vi "Array 1.vi"(8 "Error In":errorcluster) -> (0 "Error Out":errorcluster)   [LabVIEW 2014]
uses:
  <vilib>/Aledyne-TSXperts/Arduino Compatible Compiler for LabVIEW/addons/Arduino SoftwareSerial Wrapper/Arduino SoftwareSerial Wrapper.lvlib
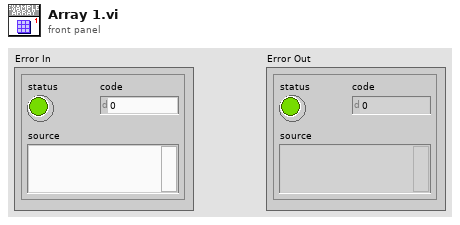
[diagram p1: front panel]
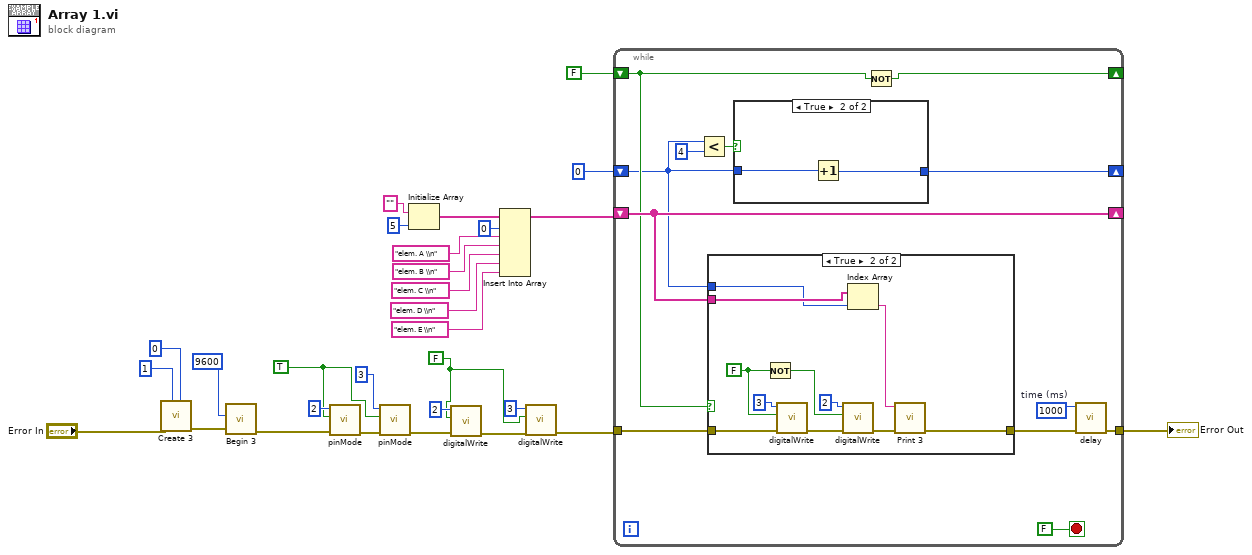
[diagram p0: block diagram]
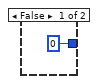
[diagram p2: hidden frame]
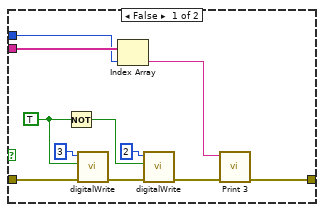
[diagram p3: hidden frame]
diagram:
  w19 = FALSE
  w26 = TRUE
  n1 = call <vilib>:"Create 3.vi"("arduino RX pin"=u8 0, "arduino TX pin"=u8 1, "Error In"="Error In") -> ("Error Out"=w16:errorcluster)  [unwired: 8 in]
  n2 = call <vilib>:"Begin 3.vi"("Error In"=w16, "Baudrate"=u16 9600) -> ("Error Out"=w14:errorcluster)  [unwired: 8 in]
  n3 = call "pinMode.vi"("Error In"=w14, "output?"=w26, "pin number"=2) -> ("Error Out"=w29:errorcluster)  [unwired: 8 in]
  n4 = call "pinMode.vi"("Error In"=w29, "output?"=w26, "pin number"=3) -> ("Error Out"=w22:errorcluster)  [unwired: 8 in]
  n5 = Initialize Array("" ("String to print"), 5 ("dimension size")) -> (w10:string[])
  n6 = call "digitalWrite.vi"("Error In"=w22, "value"=w19, "pin number"=2) -> ("Error Out"=w21:errorcluster)  [unwired: 8 in]
  n7 = Insert Into Array(array=w10, index=0, new element #1="elem. A \\n" ("String to print"), new element #2="elem. B \\n" ("String to print"), new element #3="elem. C \\n" ("String to print"), new element #4="elem. D \\n" ("String to print"), new element #5="elem. E \\n" ("String to print")) -> (w3:string[])
  n8 = call "digitalWrite.vi"("Error In"=w21, "value"=w19, "pin number"=3) -> ("Error Out"=w20:errorcluster)  [unwired: 8 in]
  n9 = while {
    tunnel: w20 -> [w39]
    tunnel: [w38] -> w25
    shift-right: [w36] -> _
    shift-left: w3 -> [w36]
    shift-right: [w33] -> _
    shift-left: 0 ("index") -> [w30]
    shift-right: [w32] -> _
    shift-left: FALSE -> [w31]
    stop <- FALSE stop-if-true
    w40 = 1000  # time (ms)
    n10 = Less?(x=w30, y=4) -> (x < y?=w35:bool)
    n11 = case shown="True" w31 {
      tunnel: w39 -> [w54 w66]
      tunnel: [w48 w59] -> w37
      tunnel: w36 -> [w47 w58]
      tunnel: w30 -> [w46 w57]
      frame False {
        w51 = TRUE
        n12 = Not(x=w51) -> (.not. x?=w52:bool)
        n13 = call "digitalWrite.vi"("Error In"=w54, "value"=w51, "pin number"=3) -> ("Error Out"=w50:errorcluster)  [unwired: 8 in]
        n14 = Index Array(array=w47, index=w46) -> (element=w45:string)
        n15 = call "digitalWrite.vi"("Error In"=w50, "value"=w52, "pin number"=2) -> ("Error Out"=w49:errorcluster)  [unwired: 8 in]
        n16 = call <vilib>:"Print 3.vi"("Error In"=w49, "String to print"=w45) -> ("Error Out"=w48:errorcluster)  [unwired: 9 in]
      }
      frame True {
        w62 = FALSE
        n17 = Not(x=w62) -> (.not. x?=w61:bool)
        n18 = call "digitalWrite.vi"("Error In"=w66, "value"=w62, "pin number"=3) -> ("Error Out"=w63:errorcluster)  [unwired: 8 in]
        n19 = call "digitalWrite.vi"("Error In"=w63, "value"=w61, "pin number"=2) -> ("Error Out"=w60:errorcluster)  [unwired: 8 in]
        n20 = Index Array(array=w58, index=w57) -> (element=w56:string)
        n21 = call <vilib>:"Print 3.vi"("Error In"=w60, "String to print"=w56) -> ("Error Out"=w59:errorcluster)  [unwired: 9 in]
      }
    }
    n22 = case shown="True" w35 {
      tunnel: [0 w43] -> w33
      tunnel: w30 -> [_ w44]
      frame False {
      }
      frame True {
        n23 = Increment(x=w44) -> (x+1=w43:i32)
      }
    }
    n24 = Not(x=w31) -> (.not. x?=w32:bool)
    n25 = call "delay.vi"("Error In"=w37, "time (ms)"=w40) -> ("Error Out"=w38:errorcluster)  [unwired: 9 in]
  }
  "Error Out" <- w25
